vi "Max Read Single.vi"(8 "error in":errorcluster, 9 "Channel Index":i32=1, 11 "Max Power Limit in":refnum<class "Power Limit.lvclass">) -> (0 "error out":errorcluster, 1 "Changed or First Call?":bool, 2 "Power Max SP":dbl, 3 "Max Power Limit out":refnum<class "Power Limit.lvclass">)   [LabVIEW 2023, in "Power Limit.lvclass"]
uses:
  Power Limit.lvclass
  Parents/Limit/Limit.lvclass
  Power Limit.lvclass/Power Limit.ctl
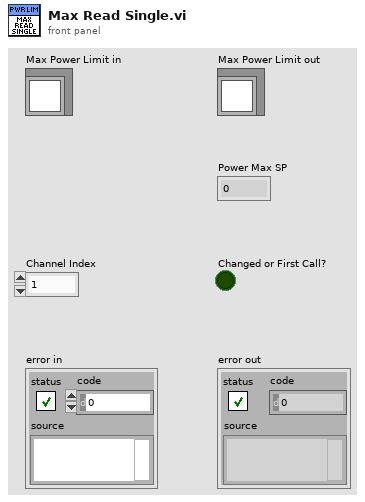
[diagram p1: front panel]
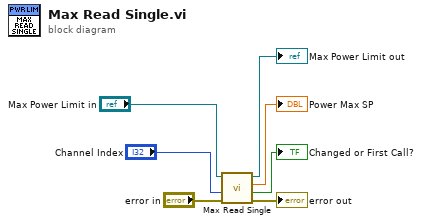
[diagram p0: block diagram]
diagram:
  n1 = call-parent "Max Read Single.vi"("error in"="error in", "Channel Index"="Channel Index", "Max Limit in"="Max Power Limit in") -> ("error out"=→"error out":errorcluster, "Changed or First Call?"=→"Changed or First Call?":bool, "Current Max Limit"=→"Power Max SP":dbl, "Max Limit out"=→"Max Power Limit out":refnum<class "Power Limit.lvclass">)  [unwired: 5 in]
